vi "Picture2Newidea.vi"() -> ()   [LabVIEW 2019]
uses:
  <vilib>/picture/picture.llb/Draw True-Color Pixmap.vi
panel:
  in  "英文1中文2":i32=2
  out "pixel center":cluster{"horizontal":i16, "vertical":i16}
  in  "Loop x":i16=10
  in  "bg color Random?":bool
  in  "Color Random?":bool
  in  "pos random":bool
  in  "text 倍數":u32=5
  in  "text":string="*"
  in  "bg color":u32(colorbox)=16777216
  in  "B/W?":bool
  out "appended path":path
  in  "Loops +1":i16
  in  "Start Ag":i16
  in  "ARC start angle":enum16{"Zero", "Random", "Loop x"}(ring)=enum."Random"
  in  "YX取大小":enum16{"取最小", "取最大", "取平均"}(ring)=enum."取平均"
  in  "輸出形狀":T1(ring)=enum."ARC"
  in  "(black)":u32(colorbox)
  in  "pen":T2={"Width"=1, "Style"=enum."Solid"}
  in  "fill?(F)":bool
  out "原來圖片大小":i32[](array[numeric])
  out "Array 5":u32[][](array[numeric])
  out "Array 4":u32[][](array[numeric])
  out "Array 3":u32[][](array[numeric])
  in  "X行融合":i32=15
  in  "Y列融合":i32=15
  out "Array":u32[][](array[numeric])
  out "Array 2":u32[][](array[numeric])
  out "output array":u32[](array[numeric])
  out "new picture":picture
  in  "輸出格式":enum16{"PNG", "JPG", "BMP"}(ring)=enum."BMP"
  in  "輸入格式":enum16{"PNG", "JPG", "BMP"}(ring)=enum."BMP"
  out "輸出圖片大小":i32[](array[numeric])
  out "original picture":picture
  # "https://ezgif.com/"
  # "選ARC>Loops+1:5>Loop x:60\n可以輸出6張PNG，再轉成GIF"
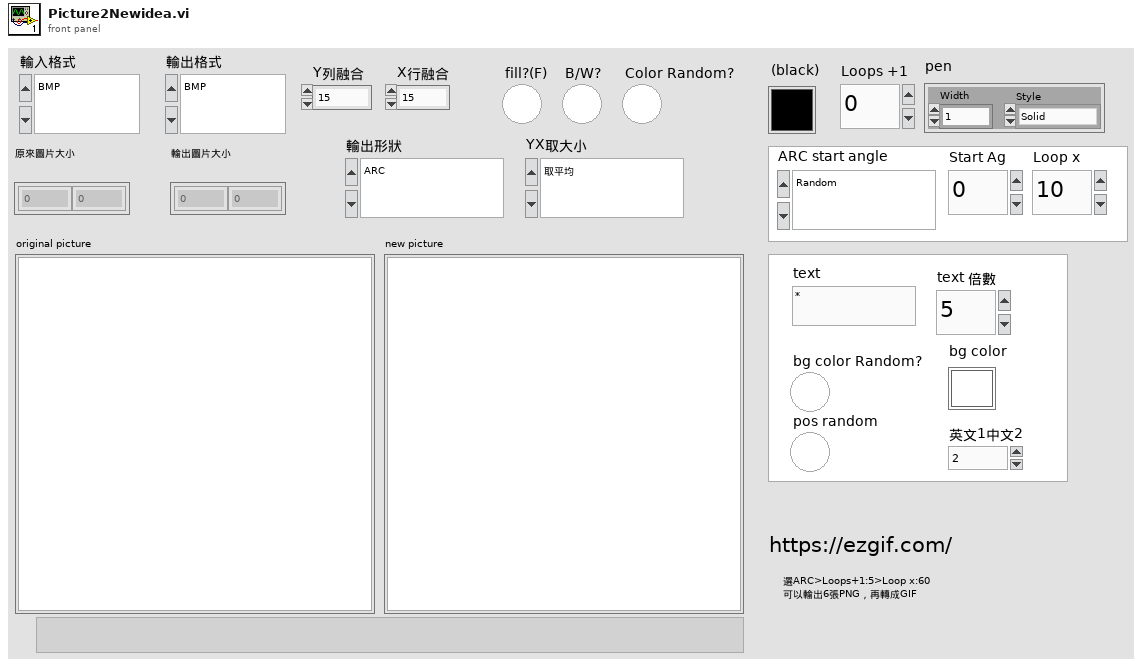
[diagram p1: front panel]
types:
  T1 = enum16{"CIRCLE", "SQUARE", "ARC", "TEXT", "LINE"}
  T2 = cluster{"Width":u16, "Style":enum32{"Solid", "Dash", "Dot", "DashDot", "DashDotDot"}}
  T3 = typedef "imagedata.ctl" = cluster{"image type":i32, "image depth":i32, "image":u8[], "mask":u8[], "colors":u32[], "Rectangle":cluster{"left":i16, "top":i16, "right":i16, "bottom":i16}}
  T4 = cluster{"horizontal":enum16{"left", "center", "right"}, "vertical":enum16{"top", "center", "bottom"}}
  T5 = cluster{"Font Name:":string, "Size":i16, "Strikeout?":bool, "Italic?":bool, "Underline?":bool, "Outline?":bool, "Shadow?":bool, "Bold?":bool}
  T6 = enum16{"User-specified Font", "Application Font", "System Font", "Dialog Font"}
  T7 = cluster{"left":i16, "top":i16, "right":i16, "bottom":i16}
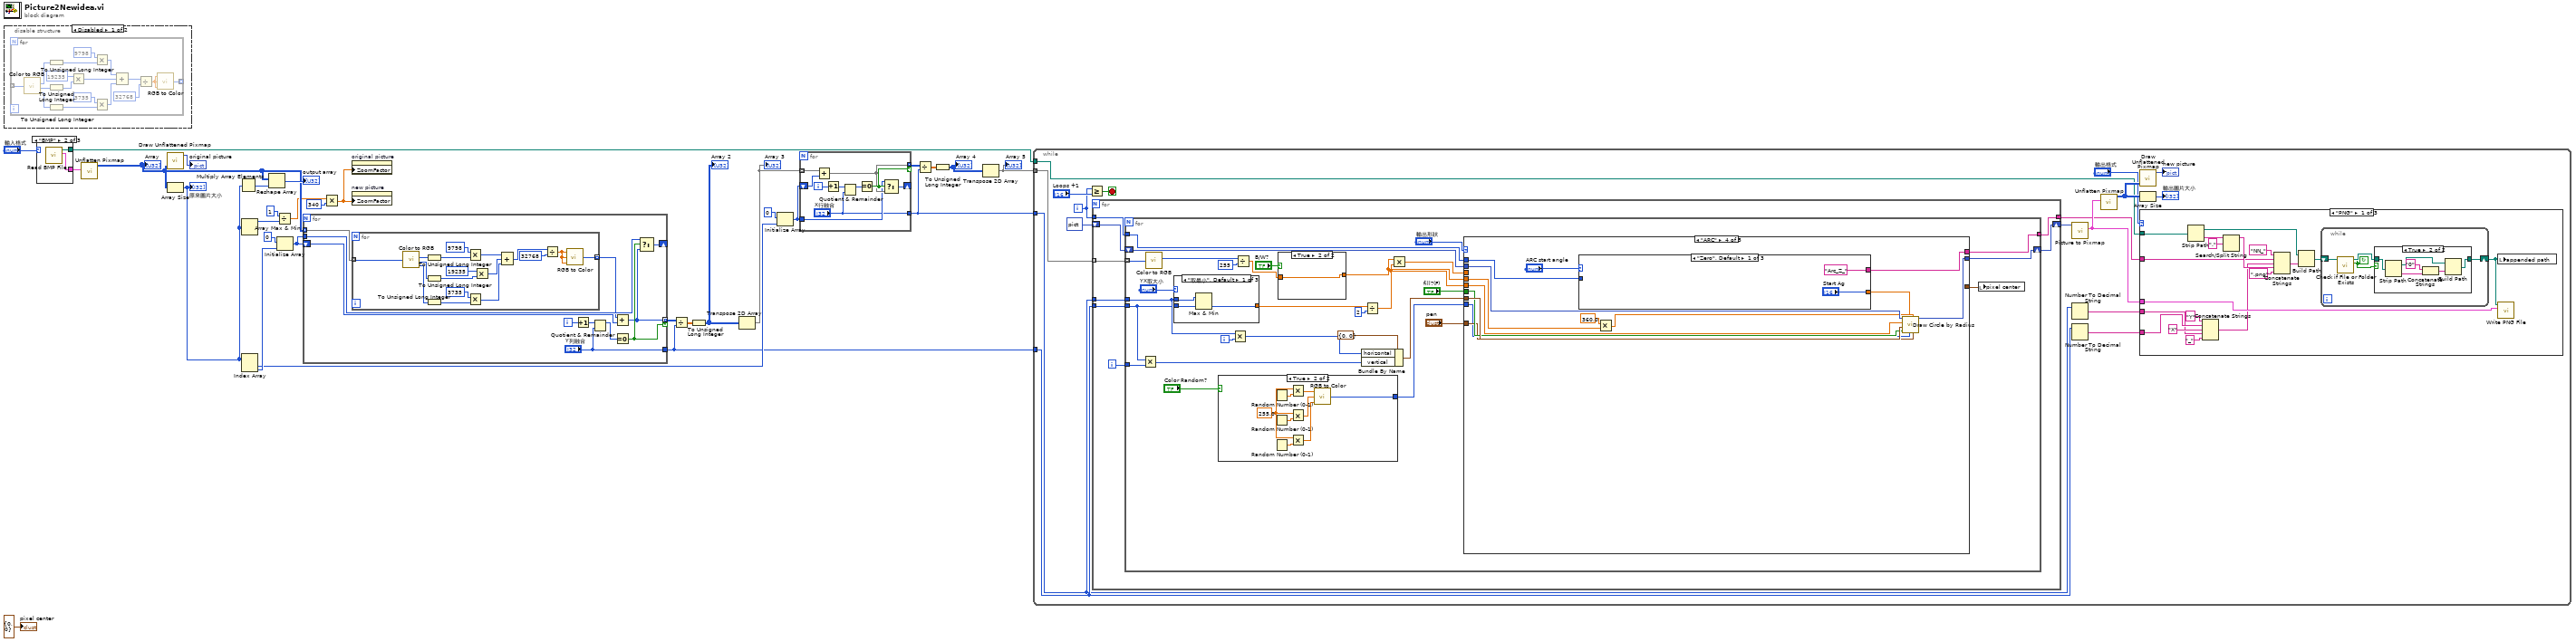
[diagram p0: block diagram]
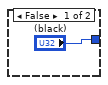
[diagram p2: hidden frame]
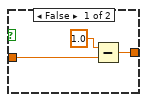
[diagram p3: hidden frame]
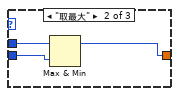
[diagram p4: hidden frame]
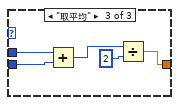
[diagram p5: hidden frame]
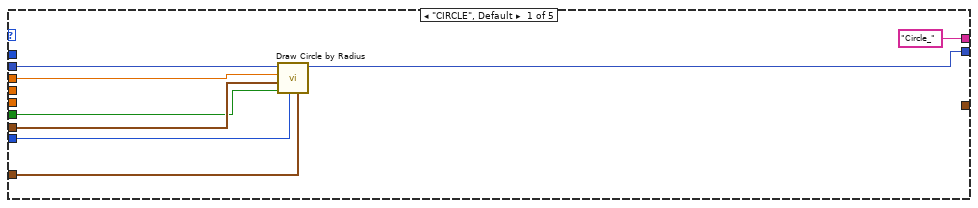
[diagram p6: hidden frame]
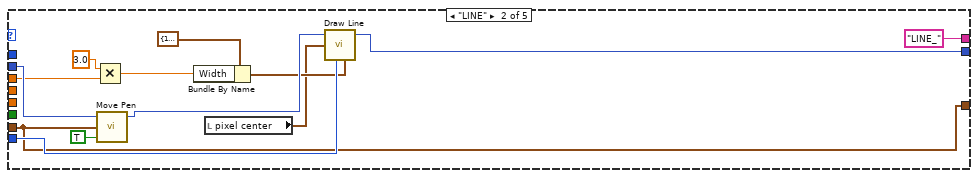
[diagram p7: hidden frame]
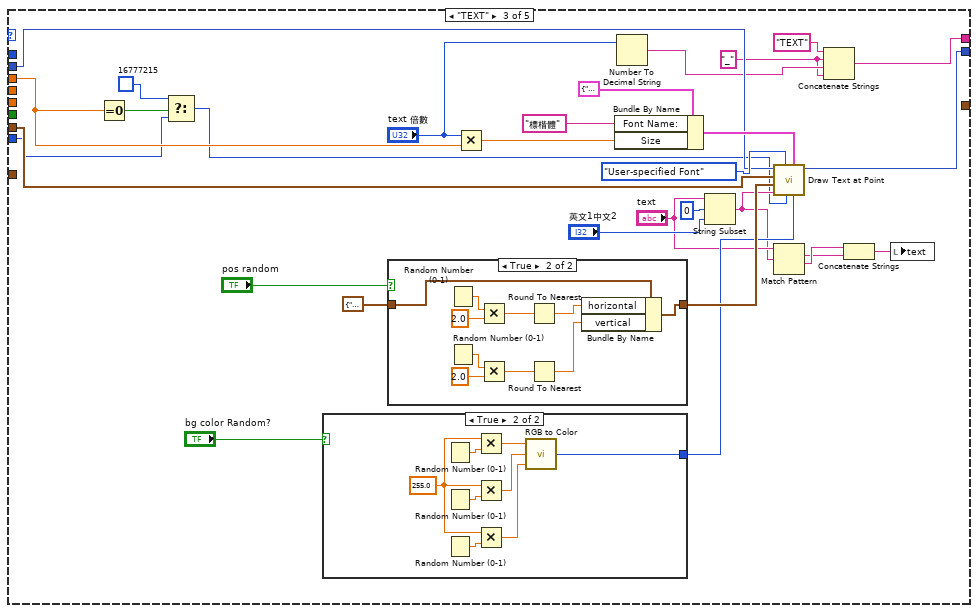
[diagram p8: hidden frame]
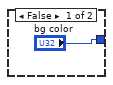
[diagram p9: hidden frame]
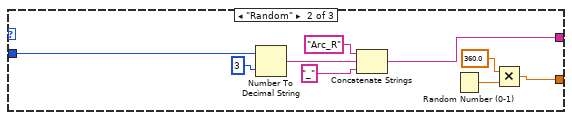
[diagram p11: hidden frame]
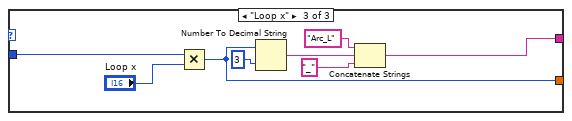
[diagram p12: hidden frame]
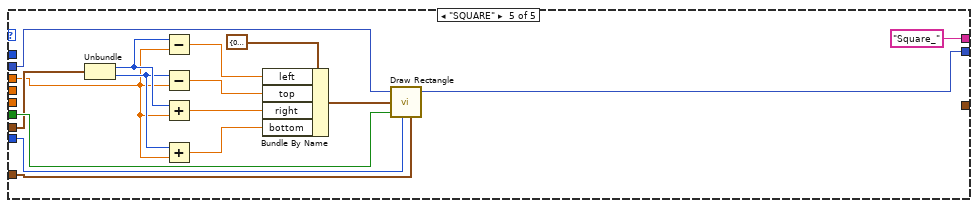
[diagram p13: hidden frame]
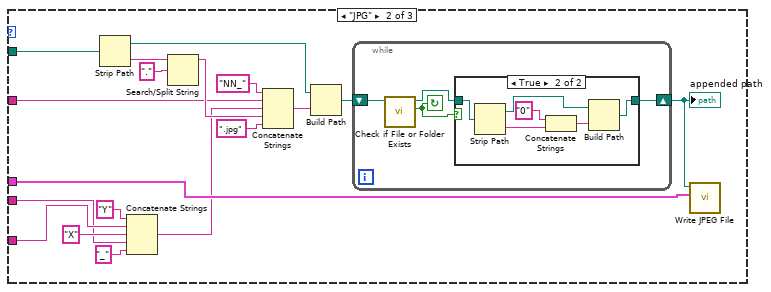
[diagram p15: hidden frame]
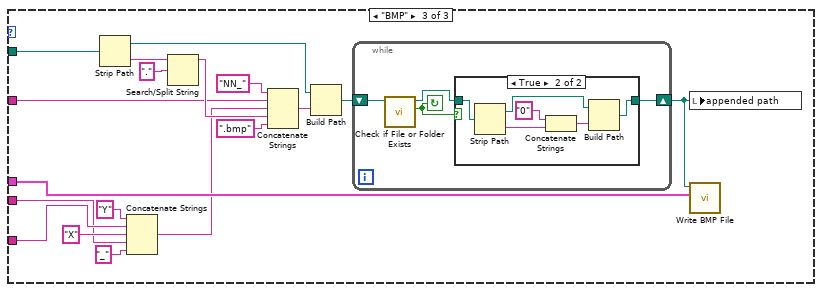
[diagram p17: hidden frame]
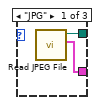
[diagram p20: hidden frame]
diagram:
  n1 = disable-structure shown="Disabled" {
    frame Disabled {
      n2 = for {
        tunnel: _ -> [w47] mode=indexing
        tunnel: [w36] -> _ mode=indexing
        n3 = call <vilib>:"Color to RGB.vi"("Color"=w47) -> ("R"=w45:u8, "G"=w44:u8, "B"=w41:u8)  [unwired: 1 out]
        n4 = To Unsigned Long Integer(number=w45) -> (unsigned 32bit integer=w34:u32)
        n5 = To Unsigned Long Integer(number=w44) -> (unsigned 32bit integer=w33:u32)
        n6 = To Unsigned Long Integer(number=w41) -> (unsigned 32bit integer=w32:u32)
        n7 = Multiply(x=u32 19235, y=w33) -> (x*y=w39:u32)
        n8 = Multiply(x=u32 9798, y=w34) -> (x*y=w40:u32)
        n9 = Multiply(x=u32 3735, y=w32) -> (x*y=w38:u32)
        n10 = Compound Arithmetic op=ADD(w40, w39, w38) -> (w35:u32)
        n11 = Divide(x=w35, y=u32 32768) -> (x/y=w31:dbl)
        n12 = call <vilib>:"RGB to Color.vi"("B"=w31, "G"=w31, "R"=w31) -> ("Color"=w36:u32)
      }
    }
    frame Enabled {
    }
  }
  n13 = case shown="\"BMP\"" "輸入格式" {
    tunnel: [w49 w51 w53] -> w30
    tunnel: [w48 w50 w52] -> w27
    frame "JPG" {
      n14 = call <vilib>:"Read JPEG File.vi"() -> ("image data"=w49:T3, "path"=w48:path)  [unwired: 9 in, 1 out]
    }
    frame "BMP" {
      n15 = call <vilib>:"Read BMP File.vi"() -> ("image data"=w51:T3, "path"=w50:path)  [unwired: 9 in, 1 out]
    }
    frame "PNG" {
      n16 = call <vilib>:"Read PNG File.vi"() -> ("image data"=w53:T3, "path"=w52:path)  [unwired: 9 in, 1 out]
    }
  }
  n17 = call <vilib>:"Unflatten Pixmap.vi"("image data"=w30) -> ("24-bit pixmap"=w24:u32[][])  [unwired: 4 in, 6 out]
  "Array" <- w24
  n18 = call-poly <vilib>:"Draw Unflattened Pixmap.vi"("data (RGB format)"=w24) -> ("new picture"=→"original picture":picture)  [unwired: 8 in]
  n19 = Array Size(array=w24) -> (size(s)=w7:i32[])
  "原來圖片大小" <- w7
  n20 = Multiply Array Elements(1:w7) -> (0:w26:i32)
  n21 = Array Max & Min(array=w7) -> (max value=w6:i32)  [unwired: 3 out]
  n22 = Index Array(array=w7) -> (element #1=w19:i32, element #2=w21:i32)  [unwired: 2 in]
  n23 = Reshape Array(w24, w26) -> (→"output array":u32[])
  n24 = Divide(x=1, y=w6) -> (x/y=w4:dbl)
  n25 = Initialize Array(u32 0, w21) -> (w22:u32[])
  n26 = for {
    tunnel: w24 -> [w60] mode=indexing
    shift-right: [w57] -> _
    shift-left: w22 -> [w64]
    tunnel: [w58] -> w16 mode=indexing if=w59
    tunnel: w22 -> [w56]
    tunnel: ["Y列融合"] -> w9
    i -> [w63]
    n27 = for {
      tunnel: w60 -> [w81] mode=indexing
      tunnel: [w70] -> w55 mode=indexing
      n28 = call <vilib>:"Color to RGB.vi"("Color"=w81) -> ("R"=w79:u8, "G"=w78:u8, "B"=w75:u8)  [unwired: 1 out]
      n29 = To Unsigned Long Integer(number=w79) -> (unsigned 32bit integer=w68:u32)
      n30 = To Unsigned Long Integer(number=w78) -> (unsigned 32bit integer=w67:u32)
      n31 = To Unsigned Long Integer(number=w75) -> (unsigned 32bit integer=w66:u32)
      n32 = Multiply(x=u32 9798, y=w68) -> (x*y=w74:u32)
      n33 = Multiply(x=u32 3735, y=w66) -> (x*y=w72:u32)
      n34 = Multiply(x=u32 19235, y=w67) -> (x*y=w73:u32)
      n35 = Compound Arithmetic op=ADD(w74, w73, w72) -> (w69:u32)
      n36 = Divide(x=w69, y=u32 32768) -> (x/y=w65:dbl)
      n37 = call <vilib>:"RGB to Color.vi"("B"=w65, "G"=w65, "R"=w65) -> ("Color"=w70:u32)
    }
    n38 = Increment(x=w63) -> (x+1=w62:i32)
    n39 = Quotient & Remainder(x=w62, y="Y列融合") -> (x-y*floor(x/y)=w61:i32)  [unwired: 1 out]
    n40 = Add(x=w55, y=w64) -> (x+y=w58:u32[])
    n41 = Equal To 0?(x=w61) -> (x = 0?=w59:bool)
    n42 = Select(t=w56, s=w59, f=w58) -> (s? t:f=w57:u32[])
  }
  n43 = Multiply(x=w4, y=340) -> (x*y=w2:dbl)
  n44 = property on="original picture" class="Pict"("ZoomFactor"=w2) -> ()  [unwired: 2 in, 2 out]
  n45 = property on="new picture" class="Pict"("ZoomFactor"=w2) -> ()  [unwired: 2 in, 2 out]
  n46 = Divide(x=w16, y=w9) -> (x/y=w15:dbl[][])
  n47 = To Unsigned Long Integer(number=w15) -> (unsigned 32bit integer=w14:u32[][])
  "Array 2" <- w14
  n48 = Transpose 2D Array(2D array=w14) -> (transposed array=w17:u32[][])
  "Array 3" <- w17
  n49 = Initialize Array(u32 0, w19) -> (w18:u32[])
  n50 = for {
    tunnel: w17 -> [w82] mode=indexing
    shift-right: [w85] -> _
    shift-left: w18 -> [w91]
    tunnel: [w86] -> w13 mode=indexing if=w87
    tunnel: w18 -> [w84]
    tunnel: ["X行融合"] -> w8
    i -> [w90]
    n51 = Add(x=w82, y=w91) -> (x+y=w86:u32[])
    n52 = Increment(x=w90) -> (x+1=w89:i32)
    n53 = Quotient & Remainder(x=w89, y="X行融合") -> (x-y*floor(x/y)=w88:i32)  [unwired: 1 out]
    n54 = Equal To 0?(x=w88) -> (x = 0?=w87:bool)
    n55 = Select(t=w84, s=w87, f=w86) -> (s? t:f=w85:u32[])
  }
  n56 = Divide(x=w13, y=w8) -> (x/y=w12:dbl[][])
  n57 = To Unsigned Long Integer(number=w12) -> (unsigned 32bit integer=w11:u32[][])
  "Array 4" <- w11
  n58 = Transpose 2D Array(2D array=w11) -> (transposed array=w10:u32[][])
  "Array 5" <- w10
  n59 = while {
    tunnel: w27 -> [w92]
    tunnel: w10 -> [w105]
    tunnel: w9 -> [w100]
    tunnel: w8 -> [w99]
    i -> [w93]
    stop <- w94 stop-if-true
    n60 = Greater Or Equal?(x=w93, y="Loops +1") -> (x >= y?=w94:bool)
    n61 = for {
      tunnel: w105 -> [w116] mode=indexing
      tunnel: w100 -> [w114]
      tunnel: w99 -> [w113]
      shift-right: [w112] -> w104
      shift-left: picture data[5B] ("new picture") -> [w111]
      tunnel: [w110] -> w101
      tunnel: w93 -> [w109]
      i -> [w115]
      n62 = for {
        tunnel: w116 -> [w145] mode=indexing
        tunnel: w115 -> [w144]
        tunnel: w114 -> [w135]
        tunnel: w113 -> [w136]
        shift-right: [w130] -> w112
        shift-left: w111 -> [w138]
        tunnel: [w125] -> w110
        tunnel: w109 -> [w121]
        i -> [w143]
        n63 = Multiply(x=w135, y=w144) -> (x*y=w139:i32)
        n64 = call <vilib>:"Color to RGB.vi"("Color"=w145) -> ("R"=w129:u8)  [unwired: 3 out]
        n65 = case shown="\"取最小\", Default" "YX取大小" {
          tunnel: w136 -> [w161 w164 w169]
          tunnel: w135 -> [w160 w163 w168]
          tunnel: [w159 w162 w165] -> w134
          frame "取最小", Default {
            n66 = Max & Min(x=w161, y=w160) -> (min(x,y)=w159:i32)  [unwired: 1 out]
          }
          frame "取最大" {
            n67 = Max & Min(x=w164, y=w163) -> (max(x,y)=w162:i32)  [unwired: 1 out]
          }
          frame "取平均" {
            n68 = Add(x=w169, y=w168) -> (x+y=w167:i32)
            n69 = Divide(x=w167, y=2) -> (x/y=w165:dbl)
          }
        }
        n70 = case shown="True" "Color Random?" {
          tunnel: ["(black)" w154] -> w119
          frame False {
          }
          frame True {
            w150 = 255.0 ("x")
            n71 = Random Number (0-1)() -> (number: 0 to 1=w153:dbl)
            n72 = Random Number (0-1)() -> (number: 0 to 1=w152:dbl)
            n73 = Random Number (0-1)() -> (number: 0 to 1=w151:dbl)
            n74 = Multiply(x=w150, y=w153) -> (x*y=w149:dbl)
            n75 = Multiply(x=w150, y=w152) -> (x*y=w148:dbl)
            n76 = Multiply(x=w150, y=w151) -> (x*y=w147:dbl)
            n77 = call <vilib>:"RGB to Color.vi"("B"=w147, "G"=w148, "R"=w149) -> ("Color"=w154:u32)
          }
        }
        n78 = Multiply(x=w136, y=w143) -> (x*y=w140:i32)
        n79 = Divide(x=w129, y=u32 255) -> (x/y=w126:dbl)
        n80 = case shown="True" "B/W?" {
          tunnel: w126 -> [w157 w158]
          tunnel: [w155 w158] -> w123
          frame False {
            n81 = Subtract(x=1.0, y=w157) -> (x-y=w155:dbl)
          }
          frame True {
          }
        }
        n82 = Bundle By Name(cluster=cluster{"horizontal":i16, "vertical":i16} {"horizontal"=0, "vertical"=0} ("pixel center"), "horizontal"=w140, "vertical"=w139) -> (w141:cluster{"horizontal":i16, "vertical":i16})
        n83 = Divide(x=w134, y=2) -> (x/y=w122:dbl)
        n84 = Multiply(x=w123, y=w122) -> (x*y=w132:dbl)
        n85 = case shown="\"ARC\"" "輸出形狀" {
          tunnel: w141 -> [w177 w182 w214 w254 w282]
          tunnel: w138 -> [w176 w188 w216 w253 w285]
          tunnel: w132 -> [w170 w180 w195 _ w275]
          tunnel: "fill?(F)" -> [w175 _ _ w252 w289]
          tunnel: [w174 w183 w215 w251 w288] -> w130
          tunnel: "pen" -> [w173 _ _ w250 w287]
          tunnel: w119 -> [w172 w186 w192 w249 w286]
          tunnel: ["Circle_" ("string") "LINE_" ("string") w210 w242 "Square_" ("string")] -> w125
          tunnel: w123 -> [_ _ _ w248 _]
          tunnel: w122 -> [_ _ _ w245 _]
          tunnel: w121 -> [_ _ _ w241 _]
          tunnel: [_ w182 _ _ _] -> w117
          frame "CIRCLE", Default {
            n86 = call <vilib>:"Draw Circle by Radius.vi"("pen"=w173, "color(black)"=w172, "fill?(F)"=w175, "pixel center"=w177, "radius"=w170, "picture"=w176) -> ("new picture"=w174:picture)  [unwired: 5 in]
          }
          frame "LINE" {
            n87 = Multiply(x=3.0, y=w180) -> (x*y=w179:dbl)
            n88 = call <vilib>:"Move Pen.vi"("absolute coordinates?(T)"=TRUE, "new position"=w182, "picture"=w188) -> ("new picture"=w189:picture)  [unwired: 2 in]
            n89 = Bundle By Name(cluster=T2 {"Width"=1, "Style"=enum."Solid"} ("pen"), "Width"=w179) -> (w184:T2)
            n90 = local read "pixel center"() -> (w181:cluster{"horizontal":i16, "vertical":i16})
            n91 = call <vilib>:"Draw Line.vi"("picture"=w189, "end point"=w181, "color(black)"=w186, "pen"=w184) -> ("new picture"=w183:picture)  [unwired: 5 in]
          }
          frame "TEXT" {
            w208 = "_" ("string")
            n92 = Equal To 0?(x=w195) -> (x = 0?=w194:bool)
            n93 = Select(t=u32 16777215 ("text color(black)"), s=w194, f=w192) -> (s? t:f=w191:u32)
            n94 = case shown="True" "bg color Random?" {
              tunnel: ["bg color" w229] -> w204
              frame False {
              }
              frame True {
                w225 = 255.0 ("x")
                n95 = Random Number (0-1)() -> (number: 0 to 1=w228:dbl)
                n96 = Random Number (0-1)() -> (number: 0 to 1=w227:dbl)
                n97 = Random Number (0-1)() -> (number: 0 to 1=w226:dbl)
                n98 = Multiply(x=w225, y=w228) -> (x*y=w224:dbl)
                n99 = Multiply(x=w225, y=w227) -> (x*y=w223:dbl)
                n100 = Multiply(x=w225, y=w226) -> (x*y=w222:dbl)
                n101 = call <vilib>:"RGB to Color.vi"("B"=w222, "G"=w223, "R"=w224) -> ("Color"=w229:u32)
              }
            }
            n102 = case shown="True" "pos random" {
              tunnel: T4 {"horizontal"=enum."center", "vertical"=enum."center"} ("alignment(left, top)") -> [w230 w234]
              tunnel: [w230 w231] -> w205
              frame False {
              }
              frame True {
                n103 = Random Number (0-1)() -> (number: 0 to 1=w240:dbl)
                n104 = Random Number (0-1)() -> (number: 0 to 1=w236:dbl)
                n105 = Multiply(x=w240, y=2.0) -> (x*y=w238:dbl)
                n106 = Multiply(x=w236, y=2.0) -> (x*y=w237:dbl)
                n107 = Round To Nearest(number=w238) -> (nearest integer value=w233:dbl)
                n108 = Round To Nearest(number=w237) -> (nearest integer value=w232:dbl)
                n109 = Bundle By Name(cluster=w234, "horizontal"=w233, "vertical"=w232) -> (w231:T4)
              }
            }
            n110 = Multiply(x="text 倍數", y=w195) -> (x*y=w213:dbl)
            n111 = Bundle By Name(cluster=T5 {"Font Name:"="", "Size"=12, "Strikeout?"=FALSE, "Italic?"=FALSE, "Underline?"=FALSE, "Outline?"=FALSE, "Shadow?"=FALSE, "Bold?"=FALSE} ("[user-specified font]"), "Font Name:"="標楷體", "Size"=w213) -> (w217:T5)
            n112 = Number To Decimal String(number="text 倍數") -> (decimal integer string=w209:string)  [unwired: 1 in]
            n113 = String Subset(string="text", offset (0)=0, length (rest)="英文1中文2") -> (substring=w196:string)
            n114 = call <vilib>:"Draw Text at Point.vi"("BG color(transparent)"=w204, "[user-specified font]"=w217, "text color(black)"=w191, "desired font(Application)"=T6."User-specified Font", "text"=w196, "alignment(left, top)"=w205, "origin"=w214, "picture"=w216) -> ("new picture"=w215:picture)  [unwired: 2 in, 1 out]
            n115 = Match Pattern(string="text", regular expression=w196) -> (match substring=w199:string, after substring=w200:string)  [unwired: 1 in, 2 out]
            n116 = Concatenate Strings("TEXT" ("string"), w208, w209, w208) -> (w210:string)
            n117 = Concatenate Strings(w200, w199) -> (w198:string)
            n118 = local write "text"(w198) -> ()
          }
          frame "ARC" {
            n119 = case shown="\"Zero\", Default" "ARC start angle" {
              tunnel: ["Start Ag" w263 w267] -> w244
              tunnel: ["Arc_Z_" ("string") w257 w272] -> w242
              tunnel: w241 -> [_ w258 w271]
              frame "Zero", Default {
              }
              frame "Random" {
                n120 = Number To Decimal String(number=w258, width (-)=i16 3) -> (decimal integer string=w260:string)
                n121 = Concatenate Strings("Arc_R" ("string"), w260, "_" ("string")) -> (w257:string)
                n122 = Random Number (0-1)() -> (number: 0 to 1=w264:dbl)
                n123 = Multiply(x=360.0, y=w264) -> (x*y=w263:dbl)
              }
              frame "Loop x" {
                n124 = Multiply(x=w271, y="Loop x") -> (x*y=w267:i32)
                n125 = Number To Decimal String(number=w267, width (-)=i16 3) -> (decimal integer string=w270:string)
                n126 = Concatenate Strings("Arc_L" ("string"), w270, "_" ("string")) -> (w272:string)
              }
            }
            n127 = Multiply(x=360.0, y=w248) -> (x*y=w246:dbl)
            n128 = call <vilib>:"Draw Circle by Radius.vi"("pen"=w250, "arc size(360)"=w246, "color(black)"=w249, "start angle(0)"=w244, "fill?(F)"=w252, "pixel center"=w254, "radius"=w245, "picture"=w253) -> ("new picture"=w251:picture)  [unwired: 3 in]
          }
          frame "SQUARE" {
            n129 = Unbundle(w282) -> ("horizontal"=w281:i16, "vertical"=w279:i16)
            n130 = Subtract(x=w281, y=w275) -> (x-y=w277:dbl)
            n131 = Subtract(x=w279, y=w275) -> (x-y=w276:dbl)
            n132 = Add(x=w281, y=w275) -> (x+y=w280:dbl)
            n133 = Add(x=w279, y=w275) -> (x+y=w278:dbl)
            n134 = Bundle By Name(cluster=T7 {"left"=0, "top"=0, "right"=0, "bottom"=0} ("rect"), "left"=w277, "top"=w276, "right"=w280, "bottom"=w278) -> (w283:T7)
            n135 = call <vilib>:"Draw Rectangle.vi"("picture"=w285, "rect"=w283, "fill?(F)"=w289, "color(black)"=w286, "pen"=w287) -> ("new picture"=w288:picture)  [unwired: 4 in]
          }
        }
        n136 = local write "pixel center"(w117) -> ()
      }
    }
    n137 = call <vilib>:"Picture to Pixmap.vi"("picture"=w104) -> ("image data"=w103:T3)  [unwired: 9 in, 1 out]
    n138 = Number To Decimal String(number=w99) -> (decimal integer string=w97:string)  [unwired: 1 in]
    n139 = Number To Decimal String(number=w100) -> (decimal integer string=w98:string)  [unwired: 1 in]
    n140 = call <vilib>:"Unflatten Pixmap.vi"("image data"=w103) -> ("24-bit pixmap"=w102:u32[][])  [unwired: 4 in, 6 out]
    n141 = call-poly <vilib>:"Draw Unflattened Pixmap.vi"("data (RGB format)"=w102) -> ("new picture"=→"new picture":picture)  [unwired: 8 in]
    n142 = Array Size(array=w102) -> (size(s)=→"輸出圖片大小":i32[])
    n143 = case shown="\"PNG\"" "輸出格式" {
      tunnel: w103 -> [w307 w336 w365]
      tunnel: w92 -> [w304 w333 w362]
      tunnel: w101 -> [w293 w322 w351]
      tunnel: w98 -> [w297 w326 w355]
      tunnel: w97 -> [w296 w325 w354]
      frame "PNG" {
        n144 = Strip Path(path=w304) -> (stripped path=w306:path, name=w303:string)
        n145 = Concatenate Strings("Y" ("string"), w297, "X" ("string"), w296, "_" ("string")) -> (w292:string)
        n146 = Search/Split String(string=w303, search string/char (-)=".") -> (substring before match=w301:string)  [unwired: 1 in, 2 out]
        n147 = Concatenate Strings("NN_" ("string"), w293, w292, w301, ".png" ("string")) -> (w305:string)
        n148 = Build Path(base path=w306, name or relative path=w305) -> (appended path=w291:path)
        n149 = while {
          shift-right: [w309] -> w290
          shift-left: w291 -> [w311]
          stop <- w308 continue-if-true
          n150 = call <vilib>:"Check if File or Folder Exists.vi"("path"=w311) -> ("file or folder exists?"=w308:bool, "dup path"=w310:path)  [unwired: 8 in, 1 out]
          n151 = case shown="True" w308 {
            tunnel: w310 -> [w312 w318]
            tunnel: [w312 w313] -> w309
            frame False {
            }
            frame True {
              n152 = Strip Path(path=w318) -> (stripped path=w317:path, name=w315:string)
              n153 = Concatenate Strings("0" ("string"), w315) -> (w316:string)
              n154 = Build Path(base path=w317, name or relative path=w316) -> (appended path=w313:path)
            }
          }
        }
        n155 = local write "appended path"(w290) -> ()
        n156 = call <vilib>:"Write PNG File.vi"("image data"=w307, "path to PNG file"=w290) -> ()  [unwired: 8 in, 2 out]
      }
      frame "JPG" {
        n157 = Strip Path(path=w333) -> (stripped path=w335:path, name=w332:string)
        n158 = Concatenate Strings("Y" ("string"), w326, "X" ("string"), w325, "_" ("string")) -> (w321:string)
        n159 = Search/Split String(string=w332, search string/char (-)=".") -> (substring before match=w330:string)  [unwired: 1 in, 2 out]
        n160 = Concatenate Strings("NN_" ("string"), w322, w321, w330, ".jpg" ("string")) -> (w334:string)
        n161 = Build Path(base path=w335, name or relative path=w334) -> (appended path=w320:path)
        n162 = while {
          shift-right: [w338] -> w319
          shift-left: w320 -> [w340]
          stop <- w337 continue-if-true
          n163 = call <vilib>:"Check if File or Folder Exists.vi"("path"=w340) -> ("file or folder exists?"=w337:bool, "dup path"=w339:path)  [unwired: 8 in, 1 out]
          n164 = case shown="True" w337 {
            tunnel: w339 -> [w341 w347]
            tunnel: [w341 w342] -> w338
            frame False {
            }
            frame True {
              n165 = Strip Path(path=w347) -> (stripped path=w346:path, name=w344:string)
              n166 = Concatenate Strings("0" ("string"), w344) -> (w345:string)
              n167 = Build Path(base path=w346, name or relative path=w345) -> (appended path=w342:path)
            }
          }
        }
        "appended path" <- w319
        n168 = call <vilib>:"Write JPEG File.vi"("image data"=w336, "path to JPEG file"=w319) -> ()  [unwired: 8 in, 2 out]
      }
      frame "BMP" {
        n169 = Strip Path(path=w362) -> (stripped path=w364:path, name=w361:string)
        n170 = Concatenate Strings("Y" ("string"), w355, "X" ("string"), w354, "_" ("string")) -> (w350:string)
        n171 = Search/Split String(string=w361, search string/char (-)=".") -> (substring before match=w359:string)  [unwired: 1 in, 2 out]
        n172 = Concatenate Strings("NN_" ("string"), w351, w350, w359, ".bmp" ("string")) -> (w363:string)
        n173 = Build Path(base path=w364, name or relative path=w363) -> (appended path=w349:path)
        n174 = while {
          shift-right: [w367] -> w348
          shift-left: w349 -> [w369]
          stop <- w366 continue-if-true
          n175 = call <vilib>:"Check if File or Folder Exists.vi"("path"=w369) -> ("file or folder exists?"=w366:bool, "dup path"=w368:path)  [unwired: 8 in, 1 out]
          n176 = case shown="True" w366 {
            tunnel: w368 -> [w370 w376]
            tunnel: [w370 w371] -> w367
            frame False {
            }
            frame True {
              n177 = Strip Path(path=w376) -> (stripped path=w375:path, name=w373:string)
              n178 = Concatenate Strings("0" ("string"), w373) -> (w374:string)
              n179 = Build Path(base path=w375, name or relative path=w374) -> (appended path=w371:path)
            }
          }
        }
        n180 = local write "appended path"(w348) -> ()
        n181 = call <vilib>:"Write BMP File.vi"("image data"=w365, "path to BMP file"=w348) -> ()  [unwired: 8 in, 2 out]
      }
    }
  }
  "pixel center" <- cluster{"horizontal":i16, "vertical":i16} {"horizontal"=0, "vertical"=0} ("pixel center")
